vi "Creation ofSubVI.vi"(0 "Signal Level":dbl(slide)=0.1 min=0.0 max=20.0 step=1.0 scale=0.0..20.0) -> ()   [LabVIEW 2014]
doc: "ITI- Session 5\nThis VI is used to generated a noisy signal where noise variability and signal level is chosen by user"
panel:
  in  "stop":bool
  in  "Noise Variability":dbl(slide)=0.1 min=0.1 max=1.0 step=0.05 scale=0.0..1.0
  out "Signal Logging":dbl(graph)
  # "Creation of SubVI"
  # "Signal Level"
  # "Noise Variability"
  # "End Program"
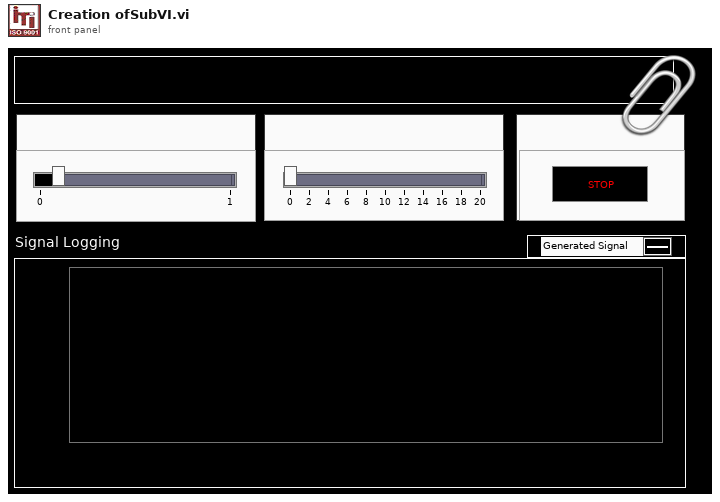
[diagram p1: front panel]
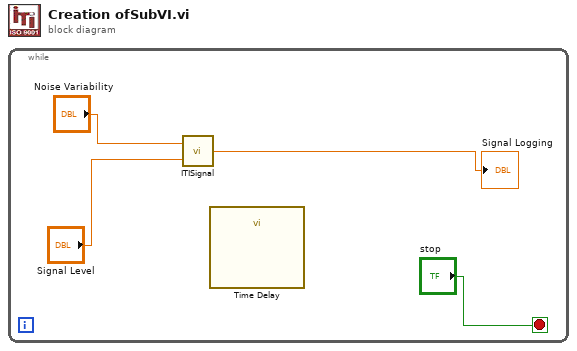
[diagram p0: block diagram]
diagram:
  n1 = while {
    stop <- "stop" stop-if-true
    n2 = call "ITISignal.vi"("SL"="Signal Level", "NV"="Noise Variability") -> ("Logging"=→"Signal Logging":dbl)
    n3 = call "Time Delay"() -> ()  [unwired: 11 in, 1 out]
  }
